vi "Get Pin Status.vi"(8 "error in (no error)":errorcluster, 9 "Pin":dbl, 10 "Port":dbl, 11 "NXP in":refnum<class "NXP.lvclass">) -> (0 "error out":errorcluster, 3 "NXP out":refnum<class "NXP.lvclass">)   [LabVIEW 2020, in "NXP.lvclass"]
uses:
  NXP.lvclass
  40c5a419-d481-45f3-adaf-3bf7732aaf60.vi
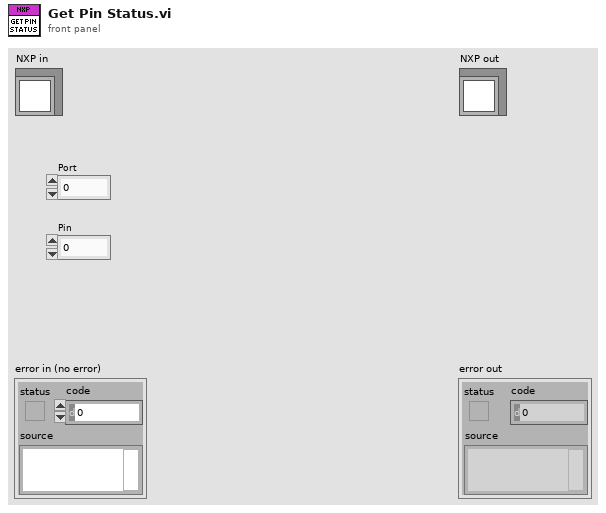
[diagram p1: front panel]
types:
  T1 = typedef "Serial device.lvclass/Brand combobox.ctl" = string
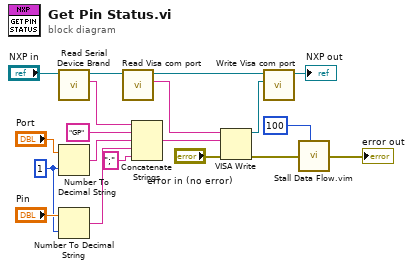
[diagram p0: block diagram]
diagram:
  w13 = i16 1 ("width (-)")
  n1 = call-dynamic "Read Serial Device Brand.vi"("Serial device in"="NXP in") -> ("Serial Device Brand"=w6:T1, "Serial device out"=w19:refnum<class "NXP.lvclass">)  [unwired: 8 in, 1 out]
  n2 = Number To Decimal String(number="Port", width (-)=w13) -> (decimal integer string=w4:string)
  n3 = Number To Decimal String(number="Pin", width (-)=w13) -> (decimal integer string=w3:string)
  n4 = call-dynamic "Read Visa com port.vi"("Serial device in"=w19) -> ("Visa com port"=w8:string, "Serial device out"=w18:refnum<class "NXP.lvclass">)  [unwired: 8 in, 1 out]
  n5 = Concatenate Strings(w6, "GP" ("string"), w4, w3, ";" ("string")) -> (w1:string)
  n6 = VISA Write(VISA resource name=w8, write buffer=w1, error in (no error)="error in (no error)") -> (VISA resource name out=w7:refnum<visa-resource-name>, error out=w12:errorcluster)  [unwired: 1 out]
  n7 = call-dynamic "Write Visa com port.vi"("Visa com port"=w7, "Serial device in"=w18) -> ("Serial device out"=→"NXP out":refnum<class "NXP.lvclass">)  [unwired: 8 in, 1 out]
  n8 = call "Stall Data Flow.vim"("value in"=w12, "milliseconds to wait"=u32 100) -> ("value out"=→"error out":errorcluster)  [unwired: 1 out]
